vi "Samples to be acquired.vi"(8 "error in (no error)":errorcluster, 10 "AOL_Globals":T1={"Imaging Protocol"=enum."AOL Z-Stack", "Number of POI"=0, "Number of Miniscans"=0, "Number of Trials"=0, "Number of Cycles "=0, "# Averaged Frames"=0, "Laser power (%)"=0, "Pockels"=0.0, "Acquisition Length (sec)"=0.0, "Fill time (us)"=0.0, "POI Dwell time (us)"=0.0, "Miniscan Dwell time per pixel (us)"=0.0, "PMT 1"=0.0, "PMT 2"=0.0, "Back Apperture"=200.0, "Frame Size"=0, "Center Frequency"=0.0, "Field of View"=0.0, "DwellTime (us)"=0.0, "Wavelength (nm)"=0.0, "Zoom"=0.0, "AOL Z"=0.0, "AOL Mode"=enum."Raster", "GridXY"=0.0, "GridZ"=0.0, "TriggerPeriod (sec)"=0.0, "Number of Pixels in Miniscan"=0, "Experiment folder path"=path "", "X centre"=0.0, "Y centre"=0.0, "Angle (degrees)"=0.0, "Plane Mode"=0, "Threshold"=[], "Regenerate Chirps"=FALSE, "Rectangle ROI length (pixels)"=0, "Rectangle ROI height (pixels)"=0, "AOD fill"=0, "Samples Wait after Trigger"=0, "StartUp Delay"=0, "Slip Cycle"=163840, "Add Cycle"=FALSE} {"Plane Mode" items=["XY Plane"]; "Frame Size" items=["100X100"=100, "128X128"=128, "200X200"=200, "256X256"=256, "512X512"=512, "1024x1024"=1024, "2048x2048"=2048]; "Back Apperture" format="%#.6g"; "Pockels" format="%#.6g"; "PMT 2" format="%#.6g"; "PMT 1" format="%#.6g"; "Angle (degrees)" format="%#.6g"; "POI Dwell time (us)" format="%#.6g"}) -> (0 "error out":errorcluster, 2 "Number of samples to be acquired (points in frame x Ch. x Av.)":u64)   [LabVIEW 2013]
uses:
  Typedefs/Controls/AOL_Globals.ctl
  Typedefs/Imaging Protocols enum.ctl
  Typedefs/Frame Size.ctl
  Typedefs/AOL modes.ctl
  Typedefs/Plane Mode.ctl
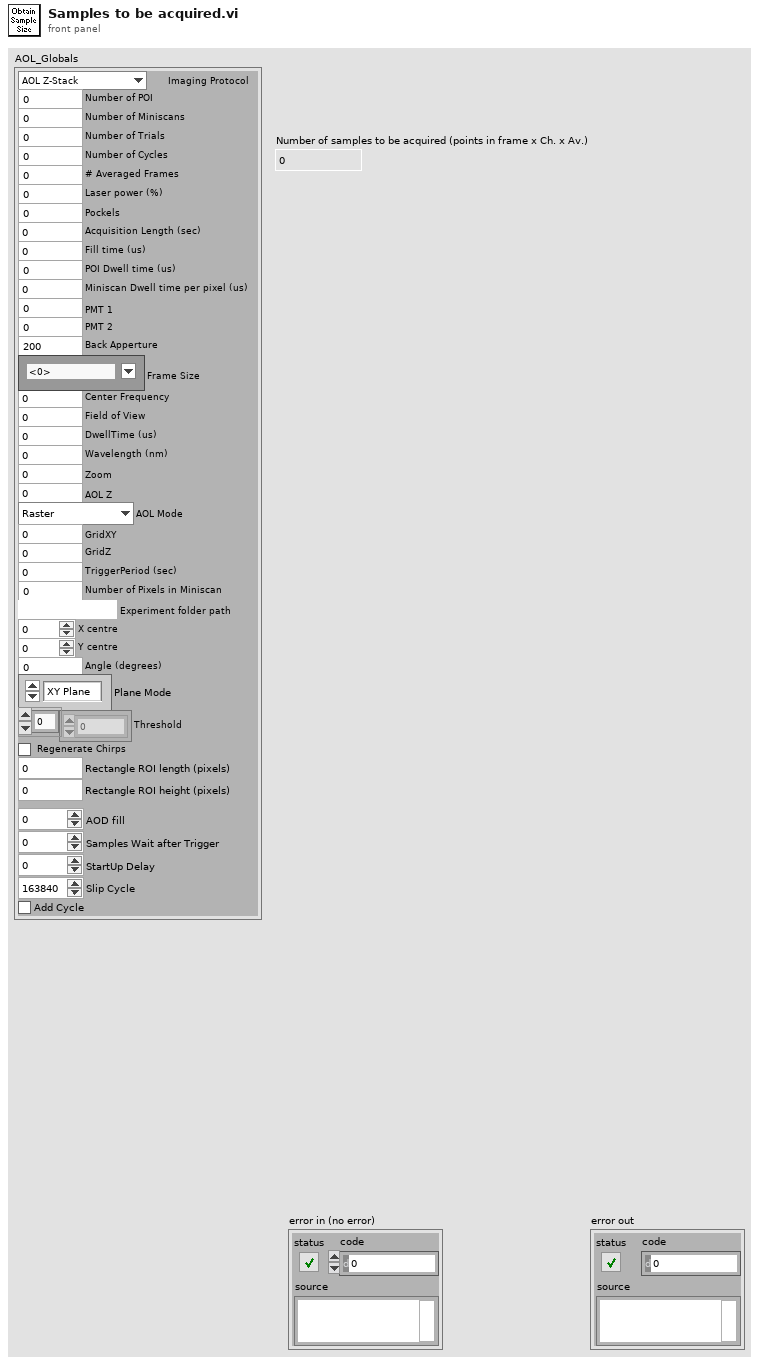
[diagram p1: front panel]
types:
  T1 = typedef "AOL_Globals.ctl" = cluster{"Imaging Protocol":T2, "Number of POI":u16, "Number of Miniscans":u16, "Number of Trials":u16, "Number of Cycles ":u64, "# Averaged Frames":u16, "Laser power (%)":u8, "Pockels":dbl, "Acquisition Length (sec)":dbl, "Fill time (us)":dbl, "POI Dwell time (us)":dbl, "Miniscan Dwell time per pixel (us)":dbl, "PMT 1":dbl, "PMT 2":dbl, "Back Apperture":dbl, "Frame Size":T3, "Center Frequency":dbl, "Field of View":dbl, "DwellTime (us)":dbl, "Wavelength (nm)":dbl, "Zoom":dbl, "AOL Z":dbl, "AOL Mode":T4, "GridXY":dbl, "GridZ":dbl, "TriggerPeriod (sec)":dbl, "Number of Pixels in Miniscan":u16, "Experiment folder path":path, "X centre":dbl, "Y centre":dbl, "Angle (degrees)":dbl, "Plane Mode":T5, "Threshold":u16[], "Regenerate Chirps":bool, "Rectangle ROI length (pixels)":u16, "Rectangle ROI height (pixels)":u16, "AOD fill":u16, "Samples Wait after Trigger":u16, "StartUp Delay":i32, "Slip Cycle":u32, "Add Cycle":bool}
  T2 = typedef "Imaging Protocols enum.ctl" = enum16{"AOL Z-Stack", "Motor Z Stack", "Functional Acquisition", "Single Plane Acquisition", "Volume Acquisition", "Live Imaging", "Live Plane Imaging", "Live Volume Imaging"}
  T3 = typedef "Frame Size.ctl" = u16
  T4 = typedef "AOL modes.ctl" = enum16{"Raster", "Structural", "Pointing", "Mini Scan", "Alignment"}
  T5 = typedef "Plane Mode.ctl" = u16
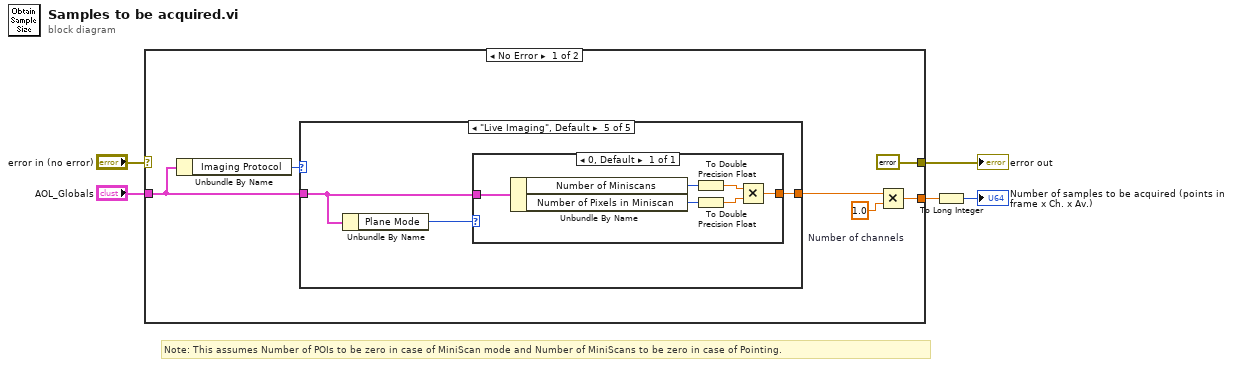
[diagram p0: block diagram]
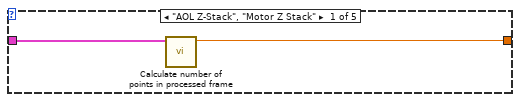
[diagram p2: hidden frame]
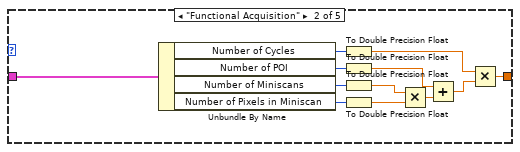
[diagram p3: hidden frame]
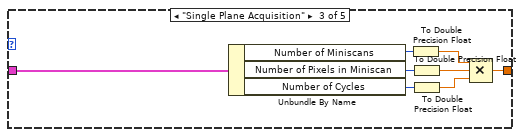
[diagram p4: hidden frame]
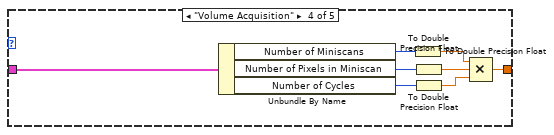
[diagram p5: hidden frame]
diagram:
  # "Note: This assumes Number of POIs to be zero in case of MiniScan mode and Number of MiniScans to be zero in case of Pointing."
  n1 = case shown="No Error" "error in (no error)" {
    selector: "error in (no error)" -> [_ w51]
    tunnel: "AOL_Globals" -> [w8 _]
    tunnel: [w7 _] -> w4
    tunnel: [errorcluster {"status"=FALSE, "code"=0, "source"=""} ("error IO") w51] -> w2
    frame No Error {
      w10 = 1.0  # Number of channels
      n2 = Unbundle By Name(w8) -> ("Imaging Protocol"=w11:T2)
      n3 = case shown="\"Live Imaging\", Default" w11 {
        tunnel: [w12 w18 w28 w36 w44] -> w9
        tunnel: w8 -> [w13 w25 w33 w41 w43]
        frame "AOL Z-Stack", "Motor Z Stack" {
          n4 = call "Calculate number of points in processed frame.vi"("AOL_Globals"=w13) -> ("Number of points in averaged frame or single frame"=w12:dbl)  [unwired: 10 in]
        }
        frame "Functional Acquisition" {
          n5 = Unbundle By Name(w25) -> ("Number of Cycles"=w24:u64, "Number of POI"=w19:u16, "Number of Miniscans"=w22:u16, "Number of Pixels in Miniscan"=w20:u16)
          n6 = To Double Precision Float(number=w24) -> (double precision float=w23:dbl)
          n7 = To Double Precision Float(number=w19) -> (double precision float=w17:dbl)
          n8 = To Double Precision Float(number=w22) -> (double precision float=w16:dbl)
          n9 = To Double Precision Float(number=w20) -> (double precision float=w15:dbl)
          n10 = Multiply(x=w16, y=w15) -> (x*y=w21:dbl)
          n11 = Add(x=w17, y=w21) -> (x+y=w14:dbl)
          n12 = Multiply(x=w23, y=w14) -> (x*y=w18:dbl)
        }
        frame "Single Plane Acquisition" {
          n13 = Unbundle By Name(w33) -> ("Number of Miniscans"=w30:u16, "Number of Pixels in Miniscan"=w31:u16, "Number of Cycles"=w32:u64)
          n14 = To Double Precision Float(number=w30) -> (double precision float=w29:dbl)
          n15 = To Double Precision Float(number=w31) -> (double precision float=w27:dbl)
          n16 = To Double Precision Float(number=w32) -> (double precision float=w26:dbl)
          n17 = Compound Arithmetic op=MULTIPLY(w29, w27, w26) -> (w28:dbl)
        }
        frame "Volume Acquisition" {
          n18 = Unbundle By Name(w41) -> ("Number of Miniscans"=w38:u16, "Number of Pixels in Miniscan"=w39:u16, "Number of Cycles"=w40:u64)
          n19 = To Double Precision Float(number=w38) -> (double precision float=w37:dbl)
          n20 = To Double Precision Float(number=w39) -> (double precision float=w35:dbl)
          n21 = To Double Precision Float(number=w40) -> (double precision float=w34:dbl)
          n22 = Compound Arithmetic op=MULTIPLY(w37, w35, w34) -> (w36:dbl)
        }
        frame "Live Imaging", Default {
          n23 = Unbundle By Name(w43) -> ("Plane Mode"=w42:T5)
          n24 = case shown="0, Default" w42 {
            tunnel: w43 -> [w46]
            tunnel: [w45] -> w44
            frame 0, Default {
              n25 = Unbundle By Name(w46) -> ("Number of Miniscans"=w50:u16, "Number of Pixels in Miniscan"=w49:u16)
              n26 = To Double Precision Float(number=w50) -> (double precision float=w48:dbl)
              n27 = To Double Precision Float(number=w49) -> (double precision float=w47:dbl)
              n28 = Multiply(x=w48, y=w47) -> (x*y=w45:dbl)
            }
          }
        }
      }
      n29 = Multiply(x=w9, y=w10) -> (x*y=w7:dbl)
    }
    frame Error {
    }
  }
  "error out" <- w2
  n30 = To Long Integer(number=w4) -> (32bit integer=→"Number of samples to be acquired (points in frame x Ch. x Av.)":i32)
